vi "test3.vi"() -> ()   [LabVIEW 2023]
uses:
  Devices/Rigol DS1054/Rigol DS1054.lvclass
  Devices/Rigol DS1054/Configurations/Voltmeter CFG/Voltmeter CFG.lvclass
  D:/git/HAL/Interfaces/IConfigure/IConfigure.lvclass
panel:
  out "Voltage":dbl
  out "error out scopes":errorcluster
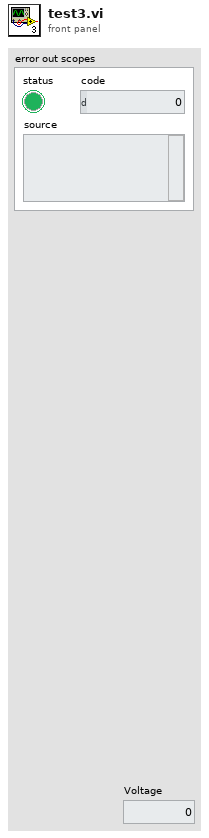
[diagram p1: front panel]
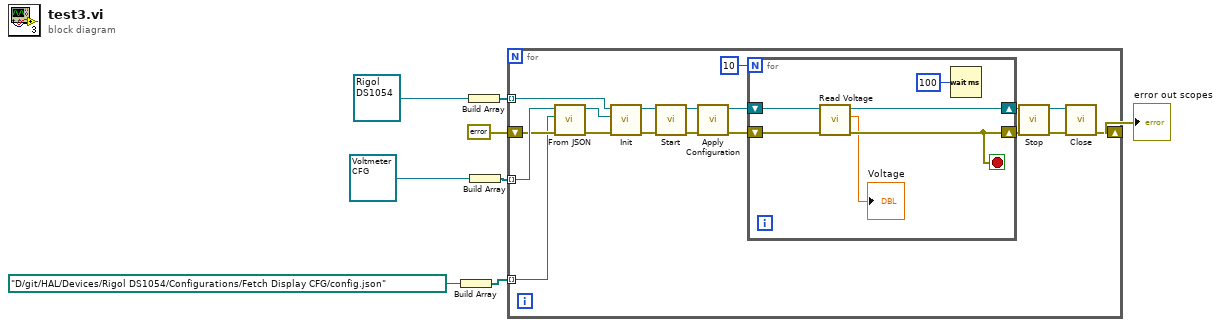
[diagram p0: block diagram]
diagram:
  n1 = Build Array(path "D:/git/HAL/Devices/Rigol DS1054/Configurations/Fetch Display CFG/config.json" ("JSON Config")) -> (w3:path[])
  n2 = Build Array(refnum<class "Rigol DS1054.lvclass"> refnum ("RIGOL DS1054.lvlib:Rigol DS1054.lvclass")) -> (w8:refnum<class "Rigol DS1054.lvclass">[])
  n3 = Build Array(refnum<class "Voltmeter CFG.lvclass"> refnum ("RIGOL DS1054Z.lvlib:Voltmeter CFG.lvclass")) -> (w7:refnum<class "Voltmeter CFG.lvclass">[])
  n4 = for {
    tunnel: w8 -> [w26] mode=indexing
    tunnel: w7 -> [w25] mode=indexing
    shift-right: [w23] -> w5
    shift-left: errorcluster {"status"=FALSE, "code"=0, "source"=""} ("error constant") -> [w21]
    tunnel: w3 -> [w19] mode=indexing
    n5 = call-dynamic "From JSON.vi"("error in (no error)"=w21, "JSON Config"=w19, "object in"=w25) -> ("error out"=w20:errorcluster, "object out"=w22:refnum<class "Voltmeter CFG.lvclass">)  [unwired: 7 in]
    n6 = call-dynamic "Init.vi"("Error In"=w20, "IConfigure"=w22, "object in"=w26) -> ("Error Out"=w24:errorcluster, "object out"=w17:refnum<class "Rigol DS1054.lvclass">)  [unwired: 7 in]
    n7 = call-dynamic "Start.vi"("Error In"=w24, "object in"=w17) -> ("Error Out"=w18:errorcluster, "object out"=w16:refnum<class "Rigol DS1054.lvclass">)  [unwired: 8 in]
    n8 = call-dynamic "Apply Configuration.vi"("error in"=w18, "Scope Base in"=w16) -> ("error out"=w12:errorcluster, "Scope Base out"=w13:refnum<class "Rigol DS1054.lvclass">)  [unwired: 8 in]
    n9 = for {
      N: 10 -> [_]
      shift-right: [w29] -> w10
      shift-left: w13 -> [w30]
      shift-right: [w28] -> w11
      shift-left: w12 -> [w28]
      stop <- w28 stop-if-true
      n10 = call-dynamic "Read Voltage.vi"("Scope Base in"=w30) -> ("Voltage"=→"Voltage":dbl, "Scope Base out"=w29:refnum<class "Rigol DS1054.lvclass">)  [unwired: 8 in, 1 out]
      n11 = Wait (ms)(milliseconds to wait=u32 100) -> ()  [unwired: 1 out]
    }
    n12 = call-dynamic "Stop.vi"("Error In"=w11, "object in"=w10) -> ("Error Out"=w15:errorcluster, "object out"=w14:refnum<class "Rigol DS1054.lvclass">)  [unwired: 8 in]
    n13 = call-dynamic "Close.vi"("Error In"=w15, "object in"=w14) -> ("Error Out"=w23:errorcluster)  [unwired: 8 in, 1 out]
  }
  "error out scopes" <- w5
